vi "CS_cRIO-PB_DP-Master_SlaveDiagData.vi"(0 "FPGA VI Reference":T1, 5 "Slave":i8, 11 "Error":errorcluster) -> (4 "FPGA VI Reference out":T1, 8 "Diagnostic data":u8[](array[numeric]) format="%.0x", 10 "Slave status":u8 format="%.0x", 15 "Error out":errorcluster)   [LabVIEW 2013, in "dynamic profibus.lvlib"]
doc: "Reads the diagnostic data of the selected DP-Slave.\n\nFPGA VI Reference:\nReference of the FPGA VI.\n\nSlave:\nPROFIBUS address of the DP-Slave. \n\nSlave status:\n0x00: DP-Slave is in DataExchange mode, input and output data are valid\n0xC3: DP-Slave is not in Data Exchange mode, input and output data are invalid, DP-Slave diagnostic data are reported in Diag data array\n0xFF: DP-Slave is in Data Exchange mode and reports ext. diagnostic data, input and output data are valid.\n\nDiagnostic data:\n\nOctet 1: StationStatus_1\nBit 7: Diag.Master_Lock\nThe DP-Slave is occupied by another DP-Master.\n\nBit 6: Diag.Prm_Fault\nThe DP-Slave received an incorrect parameter telegram, e.g. wrong length, wrong ID_Number or invalid parameters.\n\nBit 5: Diag.Invalid_Slave_Response\nAn unplausible response is received from the contacted DP-Slave.\n\nBit 4: Diag.Not_Supported\nA function has been requested which is not supported by the DP-Slave.\n\nBit 3: Diag.Ext_Diag\nA external diagnosis entry exists in the slave specific diagnosis area (Diag data). The meaning of the diagnosis is user specific and depends on the used DP-Slave model.\n\nBit 2: Diag.Cfg_Fault\nThe configuration data transmitted by the DP-Master do not comply with the DP-Slaves configuration data.\n\nBit 1: Diag.Station_Not_Ready\nThe DP-Slave is still not ready for data exchange.\n\nBit 0: Station_Non_Existent\nThe DP-Slave does not respond. \n\nOctet 2: StationStatus_2\nBit 7: Diag.Deactivated\nThe DP-Slave is determined as inactive in the DP-Slave parameter set and is excluded from the cyclic process.\n\nBit 5: Diag.Sync_Mode\nThe DP-Slave received the Sync control command.\n\nBit 4: Diag.Freeze_Mode\nThe DP-Slave received the freeze control command.\n\nBit 3: Diag.WD_On (Watchdog on)\nThe watchdog control is activated for the DP-Slave.\n\nBit 2: reserved, permanently 1\n\nBit 1: Diag.Stat_Diag (Static diagnosis)\nThe slave reports a static diagnosis\n\nBit 0: Diag.Prm_Req\nThe DP-Slave awaits a parameter telegram (e.g. after reset or wrong parameterization).\n\nOctet 3: StationStatus_3\nBit 7: Diag.Ext_Diag_Overflow\nMore diagnosis information is available than specified in Ext_Diag_Data in the slaves GS*-File.\n\nBit 0 to 6: reserved\n\nOctet 4: Diag.Master_Add\nThis octet contains the address of the DP-Master which has parameterized this DP-Slave. If the DP_Slave is not parameterized by a DP-Master, the DP-Slave inserts the address 255 in this octet.\n\nOctet 5-6: Ident_Number\nThe Ident_Number identifies the DP-Slave model and is unique for every DP-Slave.\n\nOctet 7-32: Ext_Diag_Data (extendible to 244):\nDP-Slave manufacturer specific diagnostic data.\n\nFPGA VI Reference out:\nIs a copy of the FPGA VI Reference .\n\nError in:\nPreceding error conditions. If an error has already occurred, the VI returns the value of the error in Error out.\n\nError out:\nError: TRUE if an error occurred.\nStatus: Error code\nInfo: Error description"
uses:
  dynamic profibus.lvlib
  fpga reference.ctl
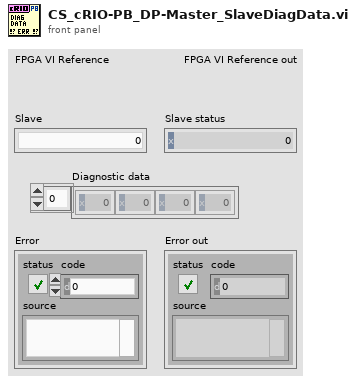
[diagram p1: front panel]
types:
  T1 = typedef "dynamic profibus.lvlib/fpga reference.ctl" = refnum<k20>
  T2 = enum16{"Start/Stop DP-Master", "Get Input Data", "Set Output Data", "Get Output Data", "Get Diagnostic Data", "Read/Write Data", "Read Diagnostic Data", "Get DPV1 Data", "Set DPV1 Data", "Read/Write DPV1 Data"}
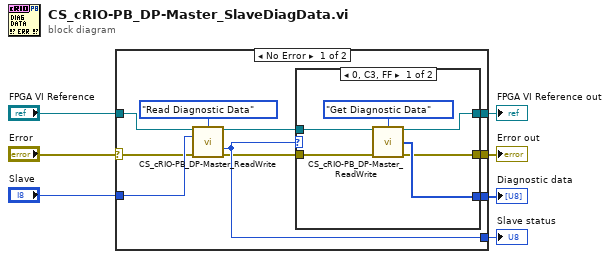
[diagram p0: block diagram]
diagram:
  n1 = case shown="No Error" "Error" {
    selector: "Error" -> [w14 w27]
    tunnel: "FPGA VI Reference" -> [w15 w26]
    tunnel: "Slave" -> [w16 _]
    tunnel: [w12 w27] -> w5
    tunnel: [w10 w26] -> w4
    tunnel: [w17 _] -> w3
    tunnel: [w9 _] -> w1
    frame No Error {
      n2 = call "CS_cRIO-PB_DP-Master_ReadWrite.vi"("FPGA VI Reference"=w15, "Mode"=T2."Read Diagnostic Data", "Slave"=w16, "Error"=w14) -> ("FPGA VI Reference out"=w11:T1, "Status"=w17:u8, "Error out"=w13:errorcluster)  [unwired: 8 in, 1 out]
      n3 = case shown="0, C3, FF" w17 {
        tunnel: w13 -> [w22 w24]
        tunnel: [w20 w24] -> w12
        tunnel: w11 -> [w23 w25]
        tunnel: [w19 w25] -> w10
        tunnel: [w21 _] -> w9
        frame 0, 195, 255 {
          n4 = call "CS_cRIO-PB_DP-Master_ReadWrite.vi"("FPGA VI Reference"=w23, "Mode"=T2."Get Diagnostic Data", "Error"=w22) -> ("FPGA VI Reference out"=w19:T1, "Data out"=w21:u8[], "Error out"=w20:errorcluster)  [unwired: 9 in, 1 out]
        }
        frame Default {
        }
      }
    }
    frame Error {
    }
  }
  "Error out" <- w5
  "FPGA VI Reference out" <- w4
  "Slave status" <- w3
  "Diagnostic data" <- w1
